vi "SpecAn Configure TxP.vi"(0 "Instrument Handle In":refnum<k21>, 1 "Selector String":string, 5 "TxP Config":T1={"Measurement Interval (s)"=0.001, "RBW (Hz)"=20000000.0, "RBW Filter Type"=2, "RRC Alpha"=0.01, "Averaging Enabled"=0, "Averaging Count"=10, "Averaging Type"=0} {"Averaging Type" items=["RMS", "Log", "Scalar", "Max", "Min"]; "Averaging Enabled" items=["False", "True"]; "RRC Alpha" format="%.3g"; "RBW Filter Type" items=["None"=5, "Gaussian"=1, "Flat"=2, "RRC"=6]; "RBW (Hz)" format="%.3p"; "Measurement Interval (s)" format="%.2p"}, 11 "error in (no error)":errorcluster) -> (4 "Instrument Handle Out":refnum<k21>, 15 "error out":errorcluster)   [LabVIEW 2019, in "RFmxSpecAn.lvlib"]
doc: "Configures common settings for the TxP measurement and selects the measurement."
uses:
  RFmxSpecAn.lvlib
  Typedefs/SpecAn TxP Configuration.ctl
  <vilib>/RFmx/SpecAn/mx/RFmxSpecAn.llb/RFmxSpecAn Select Measurement (Single).vi
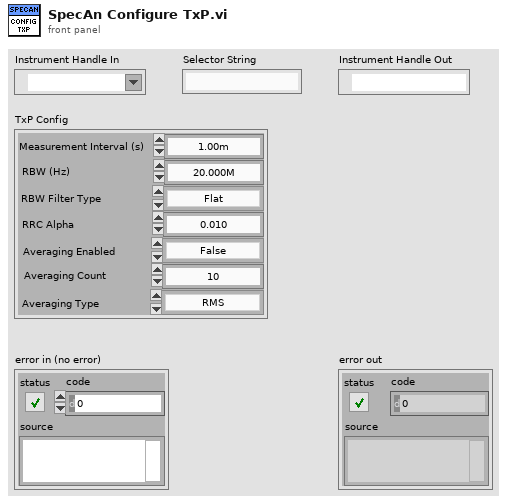
[diagram p1: front panel]
types:
  T1 = typedef "RFmxSpecAn.lvlib/SpecAn TxP Configuration.ctl" = cluster{"Measurement Interval (s)":dbl, "RBW (Hz)":dbl, "RBW Filter Type":i32, "RRC Alpha":dbl, "Averaging Enabled":i32, "Averaging Count":i32, "Averaging Type":i32}
  T2 = enum16{"ACP", "CCDF", "CHP", "FCnt", "Harmonics", "OBW", "SEM", "Spectrum", "Spur", "TXP", "AMPM", "DPD", "IQ", "IM", "NF", "PhaseNoise", "PAVT"}
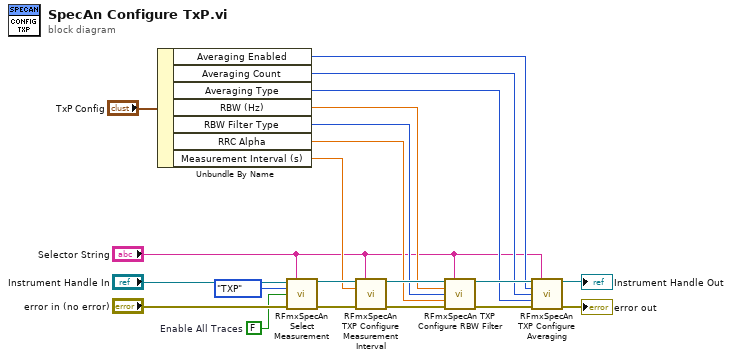
[diagram p0: block diagram]
diagram:
  w1 = FALSE  # Enable All Traces
  n1 = Unbundle By Name("TxP Config") -> ("Averaging Enabled"=w5:i32, "Averaging Count"=w6:i32, "Averaging Type"=w7:i32, "RBW (Hz)"=w8:dbl, "RBW Filter Type"=w9:i32, "RRC Alpha"=w10:dbl, "Measurement Interval (s)"=w11:dbl)
  n2 = call-poly <vilib>:"RFmxSpecAn Select Measurement.vi"("Instrument Handle In"="Instrument Handle In", "Selector String"="Selector String", "Measurement"=T2."TXP", "Enable All Traces"=w1, "error in (no error)"="error in (no error)") -> ("Instrument Handle Out"=w13:refnum<k21>, "error out"=w21:errorcluster)  [unwired: 9 in]
  n3 = call <vilib>:"RFmxSpecAn TXP Configure Measurement Interval.vi"("Instrument Handle In"=w13, "Selector String"="Selector String", "Measurement Interval (s)"=w11, "error in (no error)"=w21) -> ("Instrument Handle Out"=w20:refnum<k21>, "error out"=w19:errorcluster)  [unwired: 10 in]
  n4 = call <vilib>:"RFmxSpecAn TXP Configure RBW Filter.vi"("Instrument Handle In"=w20, "Selector String"="Selector String", "RBW (Hz)"=w8, "RBW Filter Type"=w9, "RRC Alpha"=w10, "error in (no error)"=w19) -> ("Instrument Handle Out"=w17:refnum<k21>, "error out"=w18:errorcluster)  [unwired: 8 in]
  n5 = call <vilib>:"RFmxSpecAn TXP Configure Averaging.vi"("Instrument Handle In"=w17, "Selector String"="Selector String", "Averaging Enabled"=w5, "Averaging Count"=w6, "Averaging Type"=w7, "error in (no error)"=w18) -> ("Instrument Handle Out"=→"Instrument Handle Out":refnum<k21>, "error out"=→"error out":errorcluster)  [unwired: 8 in]
